vi "DOTNET-error.vi"   [LabVIEW 2013, in "EC1000-control.lvlib" / "SM1000-control.lvclass"]
uses:
  SM1000-control.lvclass
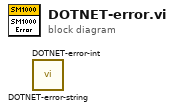
[diagram p0: block diagram]
diagram:
  n1 = call "DOTNET-error-string.vi"() -> ()  [unwired: 11 in, 1 out]
  n2 = call "DOTNET-error-int.vi"() -> ()  [unwired: 11 in, 1 out]
